vi "7.2-6.7.2-What Client.vi"() -> ()   [LabVIEW 2010]
doc: "This VI implements a client for the Named Service UDP Server.vi.\nIt connects to a service by specifying the server address and the name of the service. After sending a 'Hello' string to the server, the client receives the string sent by the server, displays the string and closes the connection.\n\n<b>Note:</b> This VI is built to work with the Named Service UDP Server.vi in UDP.llb."
uses:
  5-Forebrain/5.0-Global.vi
  7.0-Global.vi
  6-OCU Neurons/6.4-How Reporting Typedef.ctl
  6-OCU Neurons/6.0-Super Heart Beat.ctl
panel:
  out "7.5 IP-Address":string
  out "Super Heart Beat 2":T1
  out "error out":errorcluster
  out "data":T2
  out "Error":errorcluster
  in  "stop":bool
  out "Super Heart Beat":T1
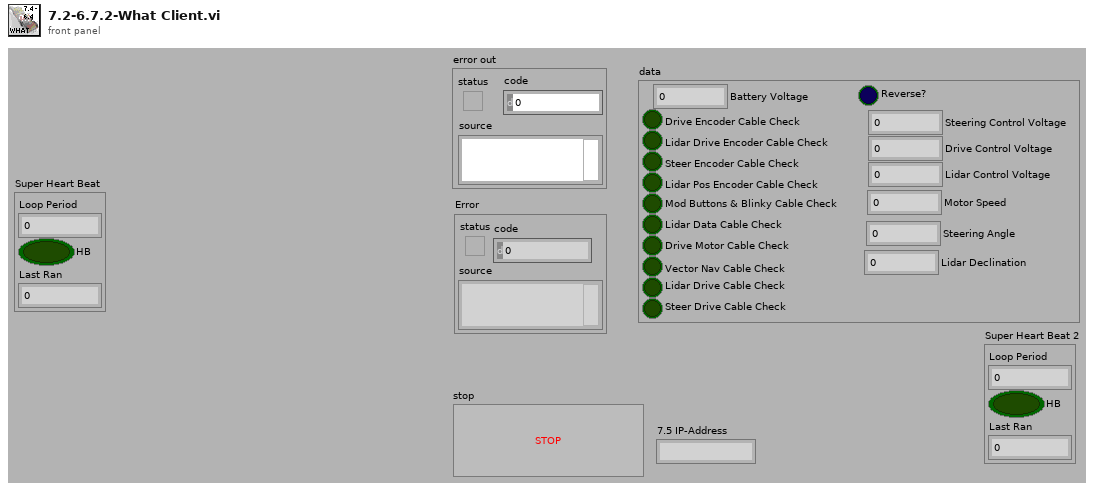
[diagram p1: front panel]
types:
  T1 = typedef "6.0-Super Heart Beat.ctl" = cluster{"Loop Period":u32, "HB":bool, "Last Ran":u32}
  T2 = typedef "6.4-How Reporting Typedef.ctl" = cluster{"Motor Speed":i32, "Lidar Declination":i32, "Steering Angle":i32, "Battery Voltage":dbl, "Drive Encoder Cable Check":bool, "Lidar Drive Encoder Cable Check":bool, "Steer Encoder Cable Check":bool, "Lidar Pos Encoder Cable Check":bool, "Mod Buttons & Blinky Cable Check":bool, "Lidar Data Cable Check":bool, "Drive Motor Cable Check":bool, "Vector Nav Cable Check":bool, "Lidar Drive Cable Check":bool, "Steer Drive Cable Check":bool, "Reverse?":bool, "Steering Control Voltage":dbl, "Drive Control Voltage":dbl, "Lidar Control Voltage":dbl}
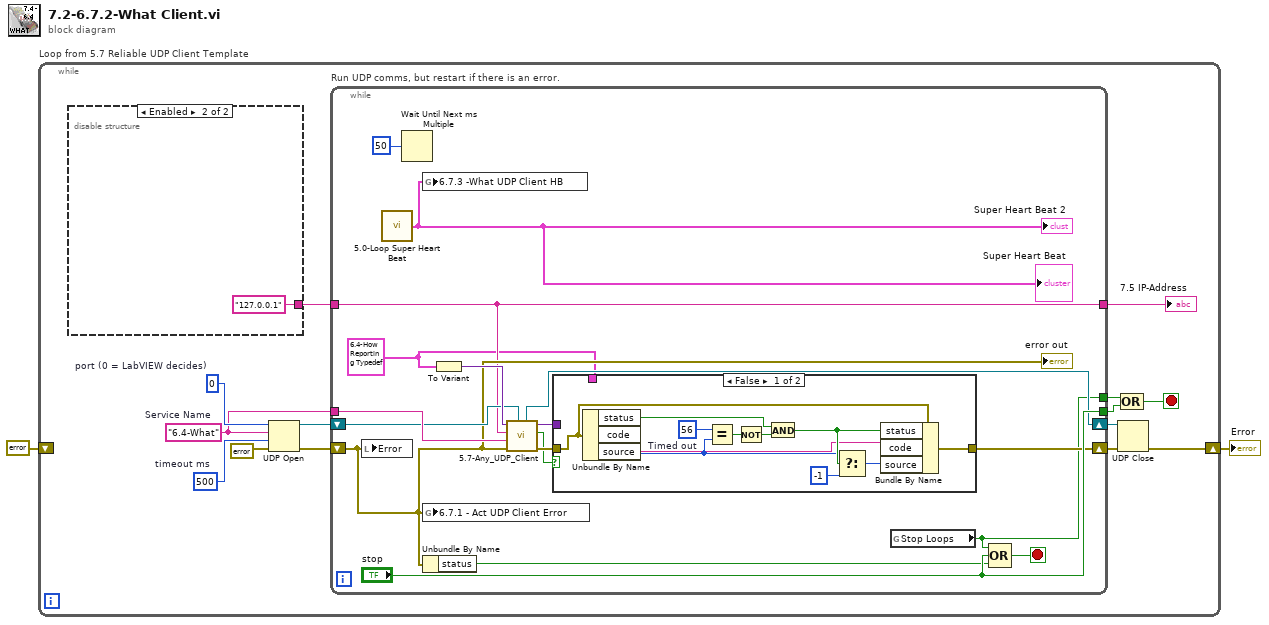
[diagram p0: block diagram]
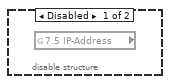
[diagram p2: hidden frame]
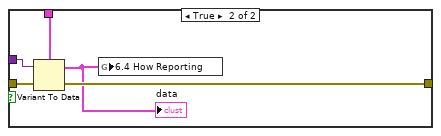
[diagram p3: hidden frame]
diagram:
  n1 = while "Loop from 5.7 Reliable UDP Client Template" {
    shift-right: [w10] -> w2
    shift-left: errorcluster {"status"=FALSE, "code"=0, "source"=""} ("error out") -> [_]
    stop <- w15 stop-if-true
    w7 = 500  # timeout ms
    w9 = u16 0  # port (0 = LabVIEW decides)
    w8 = "6.4-What"  # Service Name
    n2 = disable-structure shown="Enabled" {
      disable-tunnel: [_ "127.0.0.1" ("7.5 IP-Address")] -> w4
      frame Disabled {
        n3 = global read "7.0-Global.vi" "7.5 IP-Address"() -> ()  [unwired: 1 out]
      }
      frame Enabled {
      }
    }
    n4 = UDP Open(8:errorcluster {"status"=FALSE, "code"=0, "source"=""} ("error in (no error)"), 9:w7, 10:w8, 11:w9) -> (port=w14:refnum<k16>, 0:w12:errorcluster)  [unwired: 1 in, 1 out]
    n5 = while "Run UDP comms, but restart if there is an error." {
      tunnel: w8 -> [w32]
      tunnel: ["stop"] -> w16
      shift-right: [w26] -> w13
      shift-left: w14 -> [w27]
      shift-right: [w25] -> w11
      shift-left: w12 -> [w22]
      tunnel: [w19] -> w3
      tunnel: [w21] -> w5
      tunnel: w4 -> [w19]
      stop <- w34 stop-if-true
      w18 = T2 {"Motor Speed"=0, "Lidar Declination"=0, "Steering Angle"=0, "Battery Voltage"=0.0, "Drive Encoder Cable Check"=FALSE, "Lidar Drive Encoder Cable Check"=FALSE, "Steer Encoder Cable Check"=FALSE, "Lidar Pos Encoder Cable Check"=FALSE, "Mod Buttons & Blinky Cable Check"=FALSE, "Lidar Data Cable Check"=FALSE, "Drive Motor Cable Check"=FALSE, "Vector Nav Cable Check"=FALSE, "Lidar Drive Cable Check"=FALSE, "Steer Drive Cable Check"=FALSE, "Reverse?"=FALSE, "Steering Control Voltage"=0.0, "Drive Control Voltage"=0.0, "Lidar Control Voltage"=0.0} ("6.4 How Reporting")
      n6 = local write "Error"(w22) -> ()
      n7 = call "5.0-Loop Super Heart Beat.vi"() -> ("Super Heart Beat"=w20:T1)
      "Super Heart Beat" <- w20
      "Super Heart Beat 2" <- w20
      n8 = Wait Until Next ms Multiple(millisecond multiple=u32 50) -> ()  [unwired: 1 out]
      n9 = global write "7.0-Global.vi" "6.7.3 -What UDP Client HB"(w20) -> ()
      n10 = global write "5.0-Global.vi" "6.7.1 - Act UDP Client Error"(w22) -> ()
      n11 = Unbundle By Name(w22) -> ("status"=w28:bool)
      n12 = To Variant(anything=w18) -> (Variant=w31:variant)
      n13 = call "5.7-Any_UDP_Client.vi"("Port In"=w27, "error In"=w22, "Max Size"=w32, 10:w19, "DataTypeIn"=w31) -> ("Error Out"=w24:errorcluster, "Check Passed"=w23:bool, "DataOut"=w30:variant, "Port out"=w26:refnum<k16>)  [unwired: 3 in]
      n14 = case "Ignore Timeouts" shown="False" w23 {
        tunnel: w30 -> [_ w50]
        tunnel: w18 -> [_ w47]
        tunnel: w24 -> [w45 w49]
        tunnel: [w44 w48] -> w25
        frame False {
          w43 = 56  # Timed out
          n15 = Unbundle By Name(w45) -> ("status"=w40:bool, "code"=w38:i32, "source"=w35:string)
          n16 = Equal?(x=w43, y=w38) -> (x = y?=w42:bool)
          n17 = Not(x=w42) -> (.not. x?=w41:bool)
          n18 = And(x=w40, y=w41) -> (x .and. y?=w39:bool)
          n19 = Select(t=w38, s=w39, f=-1) -> (s? t:f=w36:i32)
          n20 = Bundle By Name(cluster=w45, "status"=w39, "code"=w36, "source"=w35) -> (w44:errorcluster)
        }
        frame True {
          n21 = Variant To Data(error in=w49, Variant=w50, type=w47) -> (error out=w48:errorcluster, data=w46:T2)
          "data" <- w46
          n22 = global write "7.0-Global.vi" "6.4 How Reporting"(w46) -> ()
        }
      }
      n23 = global read "7.0-Global.vi" "Stop Loops"() -> (w21:bool)
      n24 = Compound Arithmetic op=OR(w21, "stop", w28) -> (w34:bool)
      "error out" <- w22
    }
    "7.5 IP-Address" <- w3
    n25 = UDP Close(connection ID=w13, 8:w11) -> (error out=w10:errorcluster)  [unwired: 1 out]
    n26 = Compound Arithmetic op=OR(w5, w16) -> (w15:bool)
  }
  "Error" <- w2
